vi "補正系統時做.vi"() -> ()   [LabVIEW 2015]
uses:
  Control 9.ctl
  <vilib>/vision/Measure.llb/Edge Options.ctl
  <vilib>/vision/Measure.llb/Edge Polarity.ctl
  <vilib>/vision/NI_Vision_Development_Module.lvlib
panel:
  out "rotate":sgl
  out "Coordinate System Out":T1 {"Measurement System"."Axis Reference" items=["Direct", "Indirect"]; "Measurement System"."Angle (deg)" format="%.2f"; "Measurement System"."Origin"."Y" format="%.2f"; "Measurement System"."Origin"."X" format="%.2f"; "Reference System"."Axis Reference" items=["Direct", "Indirect"]; "Reference System"."Angle (deg)" format="%.2f"; "Reference System"."Origin"."Y" format="%.2f"; "Reference System"."Origin"."X" format="%.2f"}
  out "Intersection Point":cluster{"X":sgl, "Y":sgl} {"Y" format="%.2f"; "X" format="%.2f"}
  out "Angle":dbl format="%.2f"
  out "Y":T2
  out "X":T2
  in  "Mode":u16(ring) items=["Find Reference", "Update CoordSys"]
  in  "YOptions":T5={"Search Direction"=0, "Edge Options"={"Edge Polarity"=0, "Kernel Size"=3, "Width"=3, "Minimum Edge Strength"=10.0, "Interpolation Type"=enum."Bilinear Fixed", "Data Processing Method"=enum."Average"}, "Show Search Area"=FALSE, "Show Search Lines"=FALSE, "Show Edges Found"=FALSE, "Show Result"=TRUE, "Search Area Color"=65280, "Search Lines Color"=255, "Edge Locations Color"=16776960, "Result Color"=16711680, "Overlay Group Name"=""} {"Edge Options"."Edge Polarity" items=["All Edges", "Rising Edges", "Falling Edges"]; "Edge Options"."Minimum Edge Strength" format="%.2f"; "Edge Options"."Width" step=2; "Edge Options"."Kernel Size" step=2; "Search Direction" items=["Left to Right", "Right to Left", "Top to Bottom", "Bottom to Top"]}
  in  "XOptions":T5={"Search Direction"=0, "Edge Options"={"Edge Polarity"=0, "Kernel Size"=3, "Width"=3, "Minimum Edge Strength"=10.0, "Interpolation Type"=enum."Bilinear Fixed", "Data Processing Method"=enum."Average"}, "Show Search Area"=FALSE, "Show Search Lines"=FALSE, "Show Edges Found"=FALSE, "Show Result"=TRUE, "Search Area Color"=65280, "Search Lines Color"=255, "Edge Locations Color"=16776960, "Result Color"=16711680, "Overlay Group Name"=""} {"Edge Options"."Edge Polarity" items=["All Edges", "Rising Edges", "Falling Edges"]; "Edge Options"."Minimum Edge Strength" format="%.2f"; "Edge Options"."Width" step=2; "Edge Options"."Kernel Size" step=2; "Search Direction" items=["Left to Right", "Right to Left", "Top to Bottom", "Bottom to Top"]}
  out "element":T6
  in  "動作":bool
  in  "stop":bool
  in  "抓Y":bool
  in  "抓X":bool
  out "Image":T7(plugin-control)
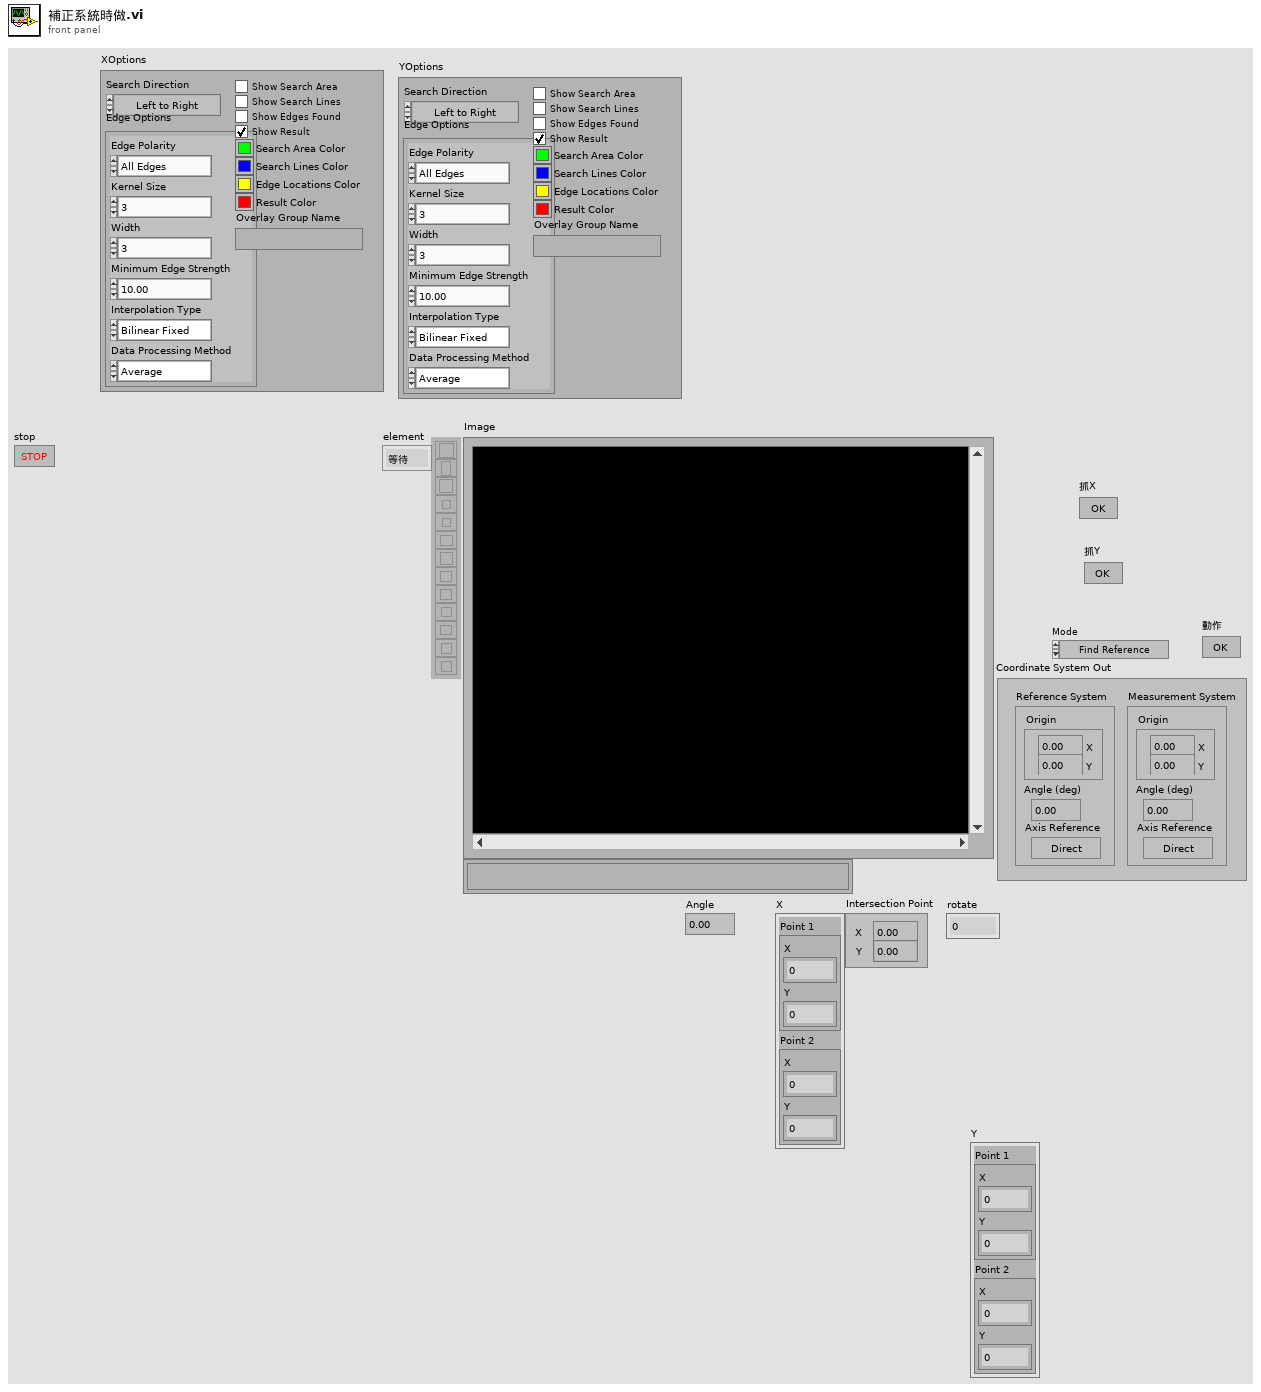
[diagram p1: front panel]
types:
  T1 = typedef "IMAQ Coordinate System" = cluster{"Reference System":cluster{"Origin":cluster{"X":sgl, "Y":sgl}, "Angle (deg)":sgl, "Axis Reference":u32}, "Measurement System":cluster{"Origin":cluster{"X":sgl, "Y":sgl}, "Angle (deg)":sgl, "Axis Reference":u32}}
  T2 = cluster{"Point 1":cluster{"X":sgl, "Y":sgl}, "Point 2":cluster{"X":sgl, "Y":sgl}}
  T3 = typedef "Edge Options.ctl" = cluster{"Edge Polarity":T4, "Kernel Size":u32, "Width":u32, "Minimum Edge Strength":sgl, "Interpolation Type":enum32{"Zero Order", "Bilinear", "Quadratic", "Cubic", "Bilinear Fixed"}, "Data Processing Method":enum32{"Average", "Median"}}
  T4 = typedef "Edge Polarity.ctl" = u32
  T5 = cluster{"Search Direction":u32, "Edge Options":T3, "Show Search Area":bool, "Show Search Lines":bool, "Show Edges Found":bool, "Show Result":bool, "Search Area Color":u32, "Search Lines Color":u32, "Edge Locations Color":u32, "Result Color":u32, "Overlay Group Name":string}
  T6 = typedef "Control 9.ctl" = enum16{"等待", "初始化", "抓X", "抓Y", "動作", "結束"}
  T7 = typedef "IMAQ Image.ctl" = refnum<image>
  T8 = typedef "Image action.ctl" = enum16{"初始化", "創造記憶體", "寫入圖片", "讀取圖片", "刪除圖片", "等待"}
  T9 = cluster{"Position":cluster{"X":sgl, "Y":sgl}, "Angle":dbl}
  T10 = cluster{"Global Rectangle":i32[], "Contours":cluster{"Contour Type":u32, "ROI Type":u32, "Points":i32[]}[]}
  T11 = cluster{"Point1 (Pixels)":cluster{"X":sgl, "Y":sgl}, "Point2 (Pixels)":cluster{"X":sgl, "Y":sgl}, "Point1 (Real-World)":cluster{"X":sgl, "Y":sgl}, "Point2 (Real-World)":cluster{"X":sgl, "Y":sgl}, "Angle (Pixel)":dbl, "Angle (Real-World)":dbl, "Score":dbl, "Straightness":dbl, "Average SNR (db)":dbl, "Calibration Valid":bool}[]
  T12 = cluster{"Point1 (Pixels)":cluster{"X":sgl, "Y":sgl}, "Point2 (Pixels)":cluster{"X":sgl, "Y":sgl}, "Point1 (Real-World)":cluster{"X":sgl, "Y":sgl}, "Point2 (Real-World)":cluster{"X":sgl, "Y":sgl}, "Angle (Pixel)":dbl, "Angle (Real-World)":dbl, "Score":dbl, "Straightness":dbl, "Average SNR (db)":dbl, "Calibration Valid":bool}
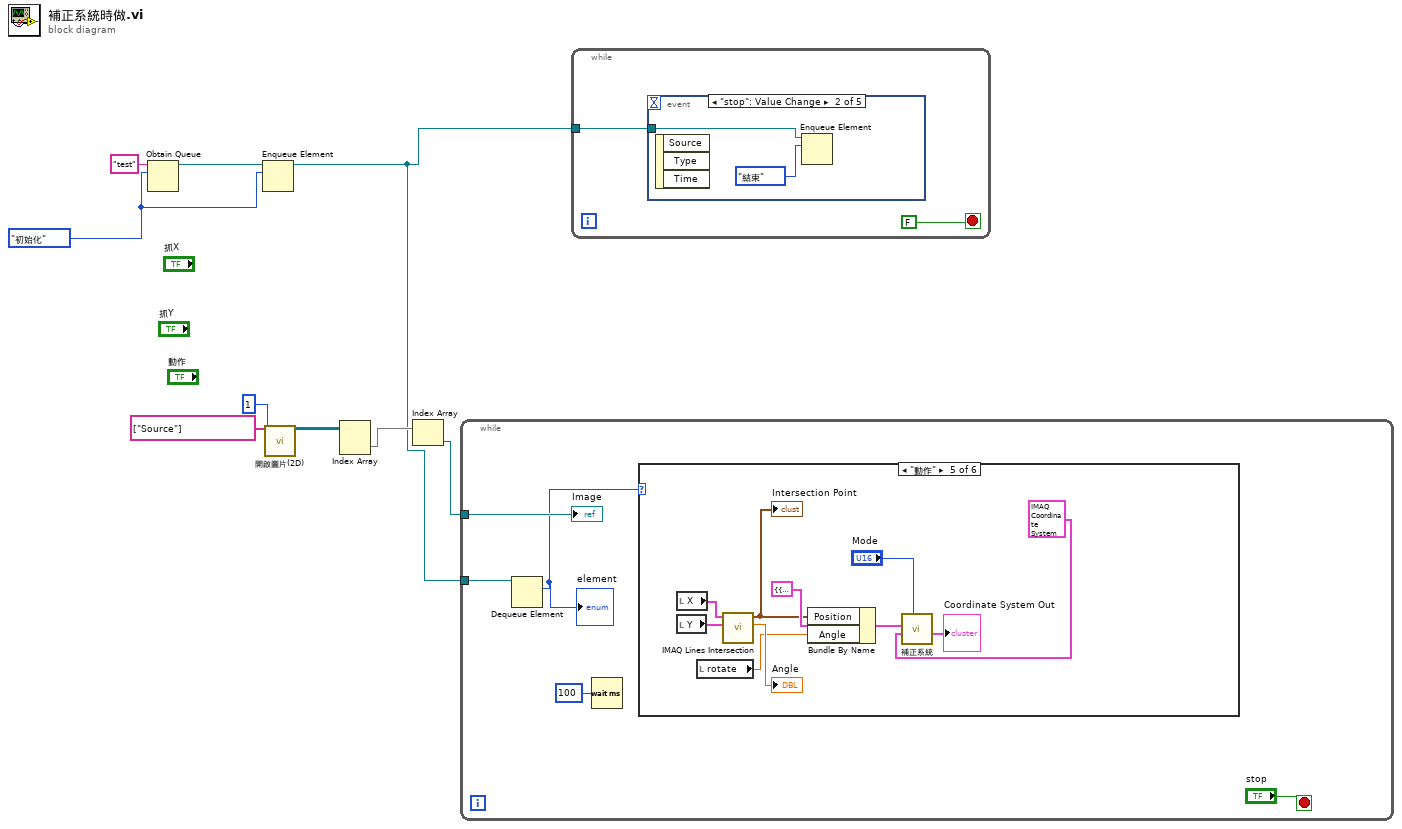
[diagram p0: block diagram]
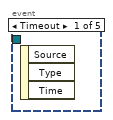
[diagram p2: hidden frame]
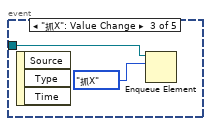
[diagram p3: hidden frame]
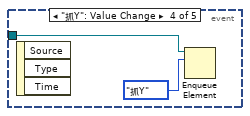
[diagram p4: hidden frame]
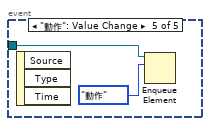
[diagram p5: hidden frame]
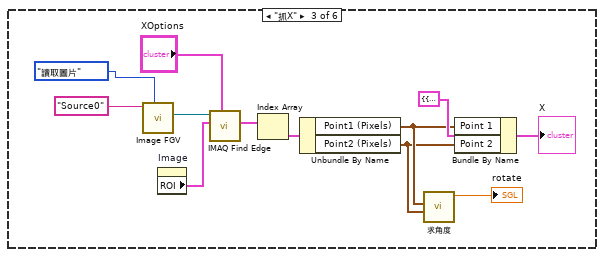
[diagram p8: hidden frame]
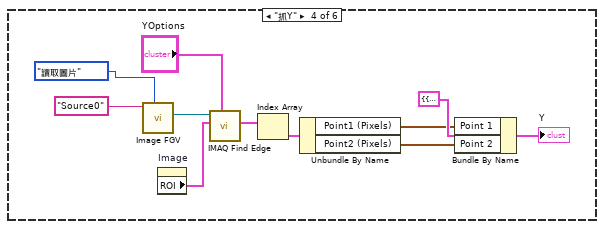
[diagram p9: hidden frame]
diagram:
  w2 = Control_9."初始化" ("Enum")
  n1 = Obtain Queue(name (unnamed)="test", element data type=w2) -> (queue out=w3:refnum<queue>)  [unwired: 3 in, 2 out]
  n2 = Enqueue Element(queue=w3, element=w2) -> (queue out=w1:refnum<queue>)  [unwired: 2 in, 2 out]
  n3 = call "開啟圖片(2D).vi"("ImageNameArray"=string[] ["Source"], "影像數量"=1) -> ("Image2DArray"=w7:T7[][])  [unwired: 9 in, 4 out]
  n4 = Index Array(array=w7) -> (element=w6:T7[])  [unwired: 2 in]
  n5 = Index Array(array=w6) -> (element=w5:T7)  [unwired: 1 in]
  n6 = while {
    tunnel: w5 -> [w14]
    tunnel: w1 -> [w11]
    stop <- "stop" stop-if-true
    n7 = Dequeue Element(queue=w11) -> (element=w10:T6)  [unwired: 2 in, 3 out]
    "element" <- w10
    n8 = Wait (ms)(milliseconds to wait=u32 100) -> ()  [unwired: 1 out]
    n9 = case shown="\"動作\"" w10 {
      frame "等待", Default {
      }
      frame "初始化" {
      }
      frame "抓X" {
        n10 = call "Image FGV.vi"("Image action"=Image_action."讀取圖片", "圖片名稱"="Source0") -> ("Image Out"=w24:T7)  [unwired: 8 in, 1 out]
        n11 = property on="Image" class="ImageControl"() -> ("ROI"=w23:T10)  [unwired: 2 in, 2 out]
        n12 = call "IMAQ Find Edge"("Options"="XOptions", "ROI Descriptor"=w23, "Image"=w24) -> ("Straight Edges"=w21:T11)  [unwired: 5 in, 3 out]
        n13 = Index Array(array=w21) -> (element=w20:T12)  [unwired: 1 in]
        n14 = Unbundle By Name(w20) -> ("Point1 (Pixels)"=w17:cluster{"X":sgl, "Y":sgl}, "Point2 (Pixels)"=w16:cluster{"X":sgl, "Y":sgl})
        n15 = call "求角度.vi"("Point 2"=w16, "Point 1"=w17) -> ("rotate"=→"rotate":sgl)  [unwired: 8 in, 1 out]
        n16 = Bundle By Name(cluster=T2 {"Point 1"={"X"=0.0, "Y"=0.0}, "Point 2"={"X"=0.0, "Y"=0.0}} ("Line 1"), "Point 1"=w17, "Point 2"=w16) -> (→"X":T2)
      }
      frame "抓Y" {
        n17 = call "Image FGV.vi"("Image action"=Image_action."讀取圖片", "圖片名稱"="Source0") -> ("Image Out"=w35:T7)  [unwired: 8 in, 1 out]
        n18 = property on="Image" class="ImageControl"() -> ("ROI"=w34:T10)  [unwired: 2 in, 2 out]
        n19 = call "IMAQ Find Edge"("Options"="YOptions", "ROI Descriptor"=w34, "Image"=w35) -> ("Straight Edges"=w27:T11)  [unwired: 5 in, 3 out]
        n20 = Index Array(array=w27) -> (element=w32:T12)  [unwired: 1 in]
        n21 = Unbundle By Name(w32) -> ("Point1 (Pixels)"=w30:cluster{"X":sgl, "Y":sgl}, "Point2 (Pixels)"=w29:cluster{"X":sgl, "Y":sgl})
        n22 = Bundle By Name(cluster=T2 {"Point 1"={"X"=0.0, "Y"=0.0}, "Point 2"={"X"=0.0, "Y"=0.0}} ("Line 1"), "Point 1"=w30, "Point 2"=w29) -> (→"Y":T2)
      }
      frame "動作" {
        n23 = local read "X"() -> (w45:T2)
        n24 = local read "Y"() -> (w46:T2)
        n25 = local read "rotate"() -> (w41:sgl)
        n26 = call "IMAQ Lines Intersection"("Line 2"=w46, "Line 1"=w45) -> ("Angle"=→"Angle":dbl, "Intersection Point"=w40:cluster{"X":sgl, "Y":sgl})  [unwired: 7 in, 1 out]
        "Intersection Point" <- w40
        n27 = Bundle By Name(cluster=T9 {"Position"={"X"=0.0, "Y"=0.0}, "Angle"=0.0} ("Cluster"), "Position"=w40, "Angle"=w41) -> (w39:T9)
        n28 = call "補正系統.vi"("element"=w39, "Coordinate System In"=T1 {"Reference System"={"Origin"={"X"=201.5, "Y"=214.5}, "Angle (deg)"=90.0, "Axis Reference"=0}, "Measurement System"={"Origin"={"X"=201.5, "Y"=214.5}, "Angle (deg)"=90.0, "Axis Reference"=0}} ("Coordinate System Out"), "Mode"="Mode") -> ("Coordinate System Out"=→"Coordinate System Out":T1)  [unwired: 5 in, 2 out]
      }
      frame "結束" {
      }
    }
    "Image" <- w14
  }
  n29 = while {
    tunnel: w1 -> [w49]
    stop <- FALSE stop-if-true
    n30 = event shown="[1] \"stop\": Value Change" {
      selector: _ -> [_ _ _ _ _]
      dyn-events: _ -> [_ _ _ _ _]
      timeout: _ -> [_ _ _ _ _]
      tunnel: w49 -> [_ w50 w52 w54 w56]
      event Timeout {
        n31 = event-data() -> ()  [unwired: 1 in, 3 out]
      }
      event "stop": Value Change {
        n32 = event-data() -> ()  [unwired: 1 in, 3 out]
        n33 = Enqueue Element(queue=w50, element=Control_9."結束" ("Enum")) -> ()  [unwired: 2 in, 3 out]
      }
      event "抓X": Value Change {
        n34 = event-data() -> ()  [unwired: 1 in, 3 out]
        n35 = Enqueue Element(queue=w52, element=Control_9."抓X" ("Enum")) -> ()  [unwired: 2 in, 3 out]
      }
      event "抓Y": Value Change {
        n36 = event-data() -> ()  [unwired: 1 in, 3 out]
        n37 = Enqueue Element(queue=w54, element=Control_9."抓Y" ("Enum")) -> ()  [unwired: 2 in, 3 out]
      }
      event "動作": Value Change {
        n38 = event-data() -> ()  [unwired: 1 in, 3 out]
        n39 = Enqueue Element(queue=w56, element=Control_9."動作" ("Enum")) -> ()  [unwired: 2 in, 3 out]
      }
    }
  }
